vi "calc_bitshift_and_scaler.vi"(8 "error in":errorcluster, 9 "ADC bits":u8=14, 10 "FIFO bits":u8=16, 11 "Cycles per pixel":u32=101) -> (0 "error out":errorcluster, 2 "Scaler":dbl, 3 "Bitshift":i8)   [LabVIEW 2011, in "Fiberscope_library.lvlib"]
uses:
  Fiberscope_library.lvlib
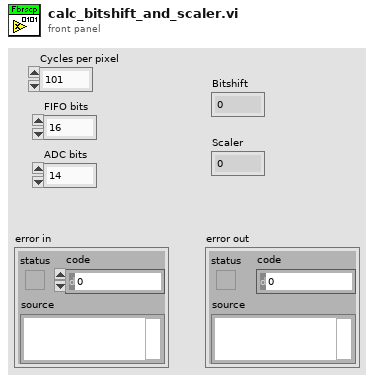
[diagram p1: front panel]
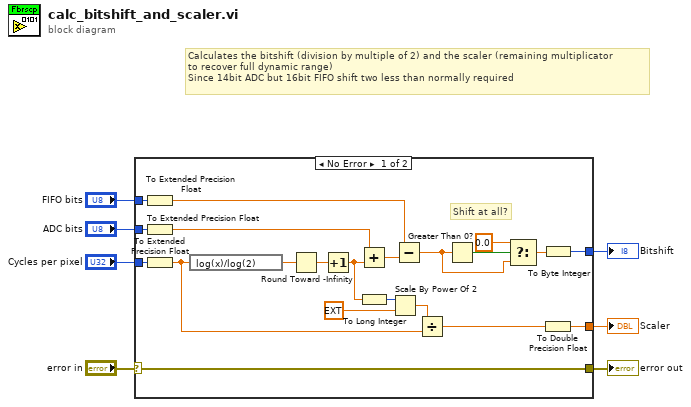
[diagram p0: block diagram]
diagram:
  # "Calculates the bitshift (division by multiple of 2) and the scaler (remaining multiplicator\nto recover full dynamic range)\nSince 14bit ADC but 16bit FIFO shift two less than normally required"
  n1 = case shown="No Error" "error in" {
    selector: "error in" -> [w8 w29]
    tunnel: "Cycles per pixel" -> [w24 _]
    tunnel: [w22 _] -> w6
    tunnel: "FIFO bits" -> [w19 _]
    tunnel: "ADC bits" -> [w17 _]
    tunnel: [w9 _] -> w3
    tunnel: [w8 w29] -> w1
    frame No Error {
      # "Shift at all?"
      n2 = To Extended Precision Float(1:w19) -> (0:w18:ext)
      n3 = To Extended Precision Float(1:w17) -> (0:w16:ext)
      n4 = To Extended Precision Float(1:w24) -> (0:w11:ext)
      n5 = expression code="log(x)/log(2)"(w11) -> (w20:ext)
      n6 = Round Toward -Infinity(1:w20) -> (0:w21:ext)
      n7 = Increment(x=w21) -> (x+1=w15:ext)
      n8 = Add(x=w16, y=w15) -> (x+y=w23:ext)
      n9 = To Long Integer(number=w15) -> (32bit integer=w14:i32)
      n10 = Scale By Power Of 2(n=w14, x=ext 1.0) -> (x*2^n=w12:ext)
      n11 = Subtract(x=w18, y=w23) -> (x-y=w27:ext)
      n12 = Divide(x=w12, y=w11) -> (x/y=w10:ext)
      n13 = Greater Than 0?(x=w27) -> (x > 0?=w25:bool)
      n14 = Select(t=0.0, s=w25, f=w27) -> (s? t:f=w28:ext)
      n15 = To Byte Integer(number=w28) -> (8bit integer=w22:i8)
      n16 = To Double Precision Float(number=w10) -> (double precision float=w9:dbl)
    }
    frame Error {
    }
  }
  "Bitshift" <- w6
  "Scaler" <- w3
  "error out" <- w1
